vi "Read stiffnessCalculated.vi"(11 "StiffnessCalculator in":refnum<class "StiffnessCalculator.lvclass">) -> (2 "stiffnessCalculated":dbl[unit] min=-888000000.0 max=888000000.0 format="%.2f", 3 "StiffnessCalculator out":refnum<class "StiffnessCalculator.lvclass">)   [LabVIEW 2015, in "StiffnessCalculator.lvclass"]
uses:
  StiffnessCalculator.lvclass
  StiffnessCalculator.lvclass/StiffnessCalculator.ctl
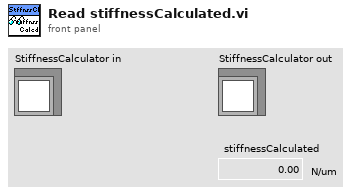
[diagram p1: front panel]
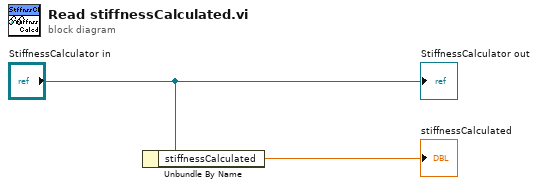
[diagram p0: block diagram]
diagram:
  n1 = Unbundle By Name("StiffnessCalculator in") -> ("stiffnessCalculated"=→"stiffnessCalculated":dbl[unit])
  "StiffnessCalculator out" <- "StiffnessCalculator in"
